vi "Launch Parallel Test.vi"(8 "error in (no error)":errorcluster, 9 "Test Complete Event":refnum<user-event>, 10 "Positions":u32[](array[numeric]), 11 "Parallel Test in":refnum<class "Parallel Test.lvclass">) -> (0 "error out":errorcluster)   [LabVIEW 2015, in "Parallel Test.lvclass"]
uses:
  Parallel Test.lvclass
  typedefs/Parallel Return -- Cluster.ctl
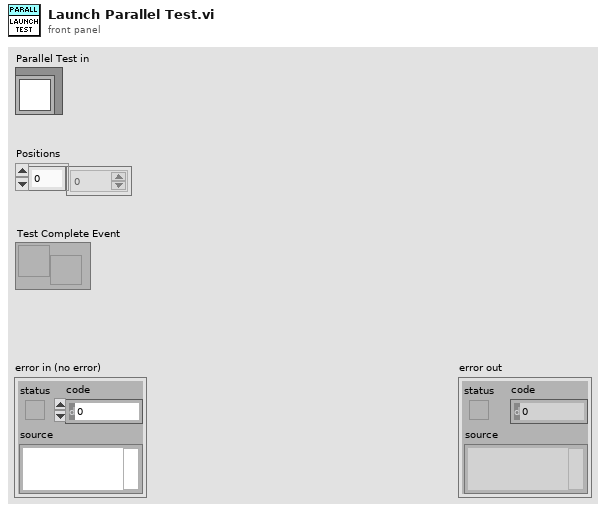
[diagram p1: front panel]
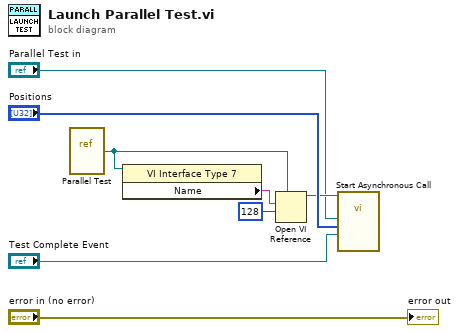
[diagram p0: block diagram]
diagram:
  n1 = vi-ref "Parallel Test.vi"() -> (w6:refnum<vi>)
  n2 = property class="VI Interface Type 7"(reference=w6) -> ("Name"=w4:string)  [unwired: 1 in, 2 out]
  n3 = Open VI Reference(type specifier VI Refnum (for type only)=w6, vi path=w4, options=128) -> (vi reference=w3:refnum<vi>)  [unwired: 3 in, 1 out]
  n4 = call-by-ref "Start Asynchronous Call"(reference=w3, "Test Complete Event"="Test Complete Event", "Positions"="Positions", "Parallel Test in"="Parallel Test in") -> ()  [unwired: 10 in, 2 out]
  "error out" <- "error in (no error)"
